vi "Get Category.vi"(8 "error in (no error)":errorcluster, 11 "CentralErrorHandlerDev editor node in":refnum<class "CentralErrorHandler editor node.lvclass">) -> (0 "error out":errorcluster, 2 "Category":string, 3 "CentralErrorHandlerDev editor node out":refnum<class "CentralErrorHandler editor node.lvclass">)   [LabVIEW 2017, in "CentralErrorHandler editor node.lvclass"]
uses:
  CentralErrorHandler editor node.lvclass
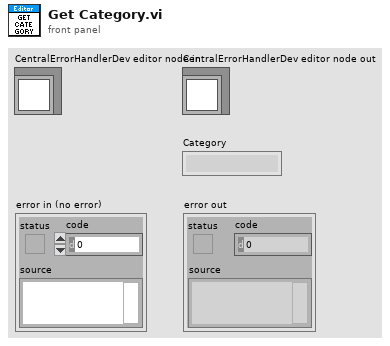
[diagram p1: front panel]
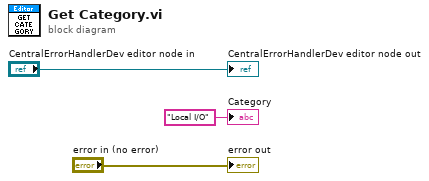
[diagram p0: block diagram]
diagram:
  "error out" <- "error in (no error)"
  "CentralErrorHandlerDev editor node out" <- "CentralErrorHandlerDev editor node in"
  "Category" <- "Local I/O" ("Category")
